vi "NIDCPower_channel_ganging - configure aperture time.vi"(7 "aperture time units":T1=1028 items=["Seconds"=1028, "Powerline Cycles"=1029], 8 "error in (no error)":errorcluster, 9 "aperture time":dbl=0.01666 format="%.6p", 11 "Ganged Session In":T2) -> (0 "error out":errorcluster, 3 "Ganged Session Out":T2)   [LabVIEW 2021]
uses:
  ctl/NIDCPower_channel_ganging - ctl - ganged session.ctl
  ctl/NIDCPower_channel_ganging - ctl - ganged config.ctl
  ctl/NIDCPower_channel_ganging - ctl - channel mode.ctl
  <instrlib>/niDCPower/nidcpower.llb/niDCPower Aperture Time Units.ctl
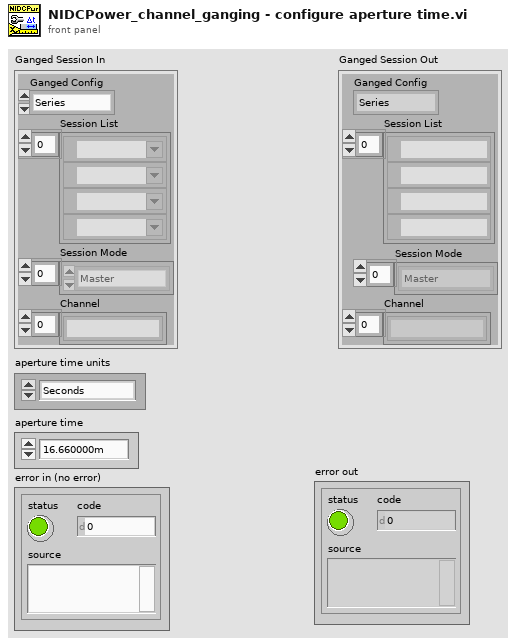
[diagram p1: front panel]
types:
  T1 = typedef "niDCPower Aperture Time Units.ctl" = i32
  T2 = typedef "NIDCPower_channel_ganging - ctl - ganged session.ctl" = cluster{"Ganged Config":T3, "Session List":refnum<k15>[], "Session Mode":T4[], "Channel":string[]}
  T3 = typedef "NIDCPower_channel_ganging - ctl - ganged config.ctl" = enum16{"Series", "Parallel", "Manual"}
  T4 = typedef "NIDCPower_channel_ganging - ctl - channel mode.ctl" = enum16{"Master", "Slave", "Slave - Inverted"}
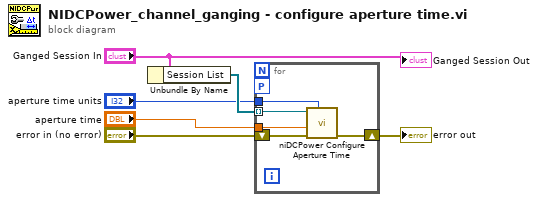
[diagram p0: block diagram]
diagram:
  n1 = Unbundle By Name("Ganged Session In") -> ("Session List"=w6:refnum<k15>[])
  n2 = for {
    workers-P: _ -> [_]
    tunnel: w6 -> [w11] mode=indexing
    shift-right: [w9] -> w3
    shift-left: "error in (no error)" -> [w10]
    tunnel: "aperture time units" -> [w8]
    tunnel: "aperture time" -> [w7]
    n3 = call <instrlib>:"niDCPower Configure Aperture Time.vi"("aperture time units"=w8, "error in (no error)"=w10, "aperture time"=w7, "instrument handle"=w11) -> ("error out"=w9:errorcluster)  [unwired: 6 in, 1 out]
  }
  "error out" <- w3
  "Ganged Session Out" <- "Ganged Session In"
